vi "GCMPlugin_IsSupportingItem.vi"(8 "error in (no error)":errorcluster, 9 "VI Reference":refnum<vi>, 10 "ProjectItem Refnum":refnum<vi>, 11 "TemplatePlugin in":refnum<class "VIWindowProperties.lvclass">) -> (0 "error out":errorcluster, 2 "IsSupportingItem":bool, 3 "TemplatePlugin out":refnum<class "VIWindowProperties.lvclass">)   [LabVIEW 2014, in "VIWindowProperties.lvlib" / "VIWindowProperties.lvclass"]
uses:
  VIWindowProperties.lvclass
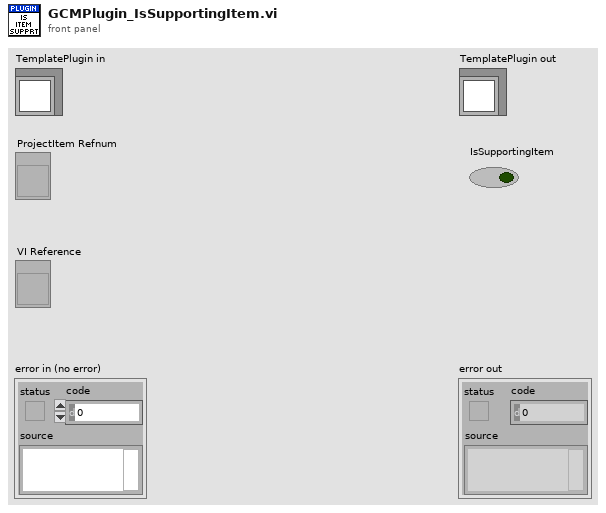
[diagram p1: front panel]
types:
  T1 = enum32{"not a control VI", "control", "typedef", "strict typedef"}
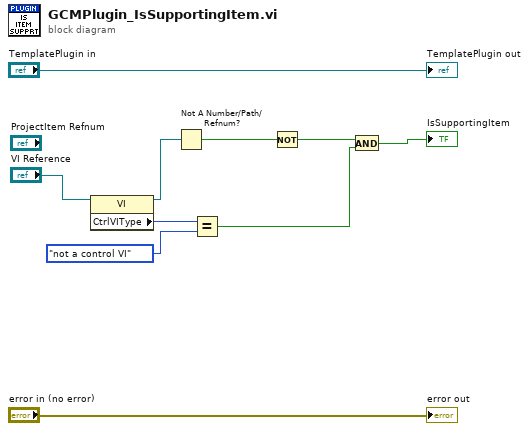
[diagram p0: block diagram]
diagram:
  n1 = property class="VI"(reference="VI Reference") -> (reference out=w5:refnum<vi>, "CtrlVIType"=w7:T1)  [unwired: 1 in, 1 out]
  n2 = Not A Number/Path/Refnum?(number/path/refnum=w5) -> (NaN/Path/Refnum?=w8:bool)
  n3 = Equal?(x=w7, y=T1."not a control VI") -> (x = y?=w1:bool)
  n4 = Not(x=w8) -> (.not. x?=w2:bool)
  n5 = And(x=w2, y=w1) -> (x .and. y?=→"IsSupportingItem":bool)
  "error out" <- "error in (no error)"
  "TemplatePlugin out" <- "TemplatePlugin in"
